vi "Stick Radius Throttle.vi"(9 "Stick Y":dbl, 11 "Stick X":dbl) -> (2 "Throttle":dbl)   [LabVIEW 2013]
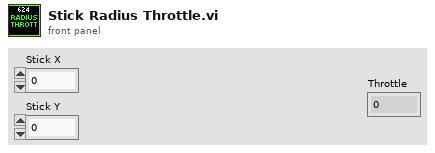
[diagram p1: front panel]
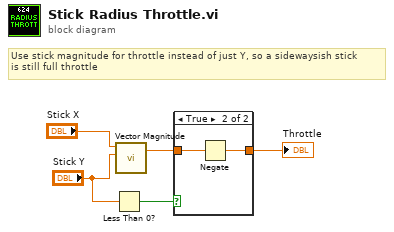
[diagram p0: block diagram]
diagram:
  # "Use stick magnitude for throttle instead of just Y, so a sidewaysish stick\nis still full throttle"
  n1 = Less Than 0?(x="Stick Y") -> (x < 0?=w3:bool)
  n2 = call "Vector Magnitude.vi"("Y"="Stick Y", "X"="Stick X") -> ("Magnitude"=w2:dbl)  [unwired: 3 in]
  n3 = case shown="True" w3 {
    tunnel: w2 -> [w6 w8]
    tunnel: [w6 w7] -> w1
    frame False {
    }
    frame True {
      n4 = Negate(x=w8) -> (-x=w7:dbl)
    }
  }
  "Throttle" <- w1
